vi "Write Single Holding Register.vi"(8 "error in (no error)":errorcluster, 9 "holding register value":u16, 10 "address":u16, 11 "Modbus master in":refnum<class "Modbus Master.lvclass">) -> (0 "error out":errorcluster, 3 "Modbus master out":refnum<class "Modbus Master.lvclass">)   [LabVIEW 2018, in "Modbus Master.lvclass"]
doc: "Writes a value to a single holding register."
uses:
  Modbus Master.lvclass
  C:/Program Files (x86)/National Instruments/LabVIEW 2018/vi.lib/Modbus/subvis/Modbus API/Modbus API.lvclass
  Modbus API.lvclass/Modbus API.ctl
  Modbus Master.lvclass/Modbus Master.ctl
  Network Master.lvclass
  C:/Program Files (x86)/National Instruments/LabVIEW 2018/vi.lib/Modbus/subvis/Protocol/Interfaces/Network Protocol/Network Protocol.lvclass
  Transmission Data Unit.lvclass
  Master Function Definition.lvlib
  Modbus API.lvclass
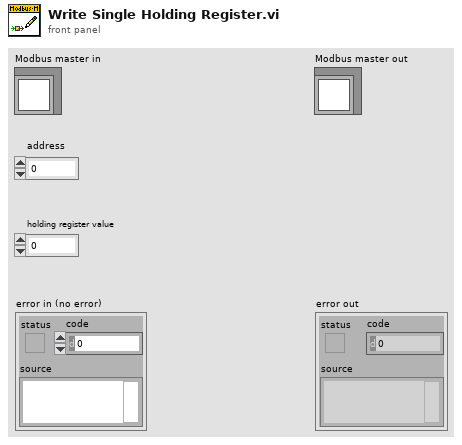
[diagram p1: front panel]
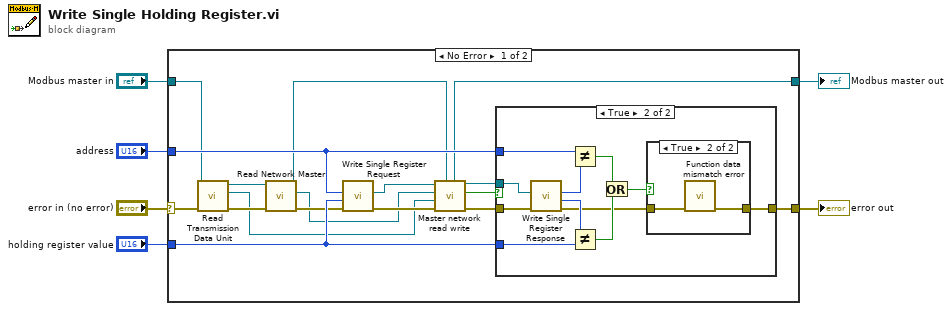
[diagram p0: block diagram]
diagram:
  n1 = case shown="No Error" "error in (no error)" {
    selector: "error in (no error)" -> [w8 w39]
    tunnel: "Modbus master in" -> [w7 w40]
    tunnel: [w16 w40] -> w4
    tunnel: [w22 w39] -> w3
    tunnel: "address" -> [w21 _]
    tunnel: "holding register value" -> [w20 _]
    frame No Error {
      n2 = call "Read Transmission Data Unit.vi"("error in (no error)"=w8, "Modbus instance in"=w7) -> ("error out"=w14:errorcluster, "transmission data unit"=w11:refnum<class "Transmission Data Unit.lvclass">, "Modbus instance out"=w15:refnum<class "Modbus Master.lvclass">)  [unwired: 7 in]
      n3 = call "Read Network Master.vi"("error in (no error)"=w14, "Modbus master in"=w15) -> ("error out"=w13:errorcluster, "network master"=w10:refnum<class "Network Master.lvclass">, "Modbus master out"=w12:refnum<class "Modbus Master.lvclass">)  [unwired: 7 in]
      n4 = call "Write Single Register Request.vi"("error in (no error)"=w13, "register value"=w20, "starting address"=w21) -> ("error out"=w23:errorcluster, "Modbus data unit out"=w18:refnum<class "Modbus Data Unit (PDU).lvclass">)  [unwired: 7 in]
      n5 = call "Master network read write.vi"("Modbus master in"=w12, "error in (no error)"=w23, "transmission data unit in"=w11, "network master in"=w10, "Modbus data unit in"=w18) -> ("error out"=w19:errorcluster, "PDU valid?"=w9:bool, "Modbus data unit out"=w17:refnum<class "Modbus Data Unit (PDU).lvclass">, "Modbus master out"=w16:refnum<class "Modbus Master.lvclass">)  [unwired: 3 in]
      n6 = case shown="True" w9 {
        tunnel: [w24 w32] -> w22
        tunnel: w21 -> [_ w26]
        tunnel: w20 -> [_ w31]
        tunnel: w19 -> [w24 w29]
        tunnel: w17 -> [_ w28]
        frame False {
        }
        frame True {
          n7 = call "Write Single Register Response.vi"("error in (no error)"=w29, "Modbus data unit in"=w28) -> ("error out"=w27:errorcluster, "number of coils"=w30:u16, "address"=w25:u16)  [unwired: 7 in]
          n8 = Not Equal?(x=w26, y=w25) -> (x != y?=w34:bool)
          n9 = Not Equal?(x=w30, y=w31) -> (x != y?=w35:bool)
          n10 = Or(x=w34, y=w35) -> (x .or. y?=w33:bool)
          n11 = case shown="True" w33 {
            tunnel: [w36 w38] -> w32
            tunnel: w27 -> [w36 w37]
            frame False {
            }
            frame True {
              n12 = call "Function data mismatch error.vi"("error in (no error)"=w37) -> ("error out"=w38:errorcluster)  [unwired: 10 in]
            }
          }
        }
      }
    }
    frame Error {
    }
  }
  "error out" <- w3
  "Modbus master out" <- w4
